vi "Layer Parameters Write Low Level.vi"(8 "Error In":errorcluster, 10 "Layer Information Cluster":T2 {"Deposition Method" items=["Front Electrode", "Electron Transport Layer", "Active Layer", "Hole Transport Layer", "Back Electrode", "Custom Layer"]; "Layer Type" items=["Front Electrode", "Electron Transport Layer", "Active Layer", "Hole Transport Layer", "Back Electrode", "Custom Layer"]}, 11 "Database Full Information In":T1 {"Database Write Information"."Layer Information Array"."Deposition Method" items=["Blade Coating", "Spin Coating", "Thermal Evaporation", "E-Beam Evaporation", "Sputtering", "Drop Casting", "Dip Coating", "Pulsed Laser Deposition", "Chemival Vapour Deposition", "Atomic Layer Deposition", "Spray Coating", "Screen Printing", "Electroplating", "Molecular Beam Epitaxy", "Custom Deposition"]; "Database Write Information"."Layer Information Array"."Layer Type" items=["Front Electrode", "Electron Transport Layer", "Active Layer", "Hole Transport Layer", "Back Electrode", "Custom Layer"]}) -> (0 "Error Out":errorcluster)   [LabVIEW 2020]
uses:
  Data Clusters/Layer Information Cluster.ctl
  Data Clusters/Database Information.ctl
  <vilib>/addons/database/Connection.llb/Conn ObjectReference.ctl
  <vilib>/addons/database/NI_Database_API.lvlib
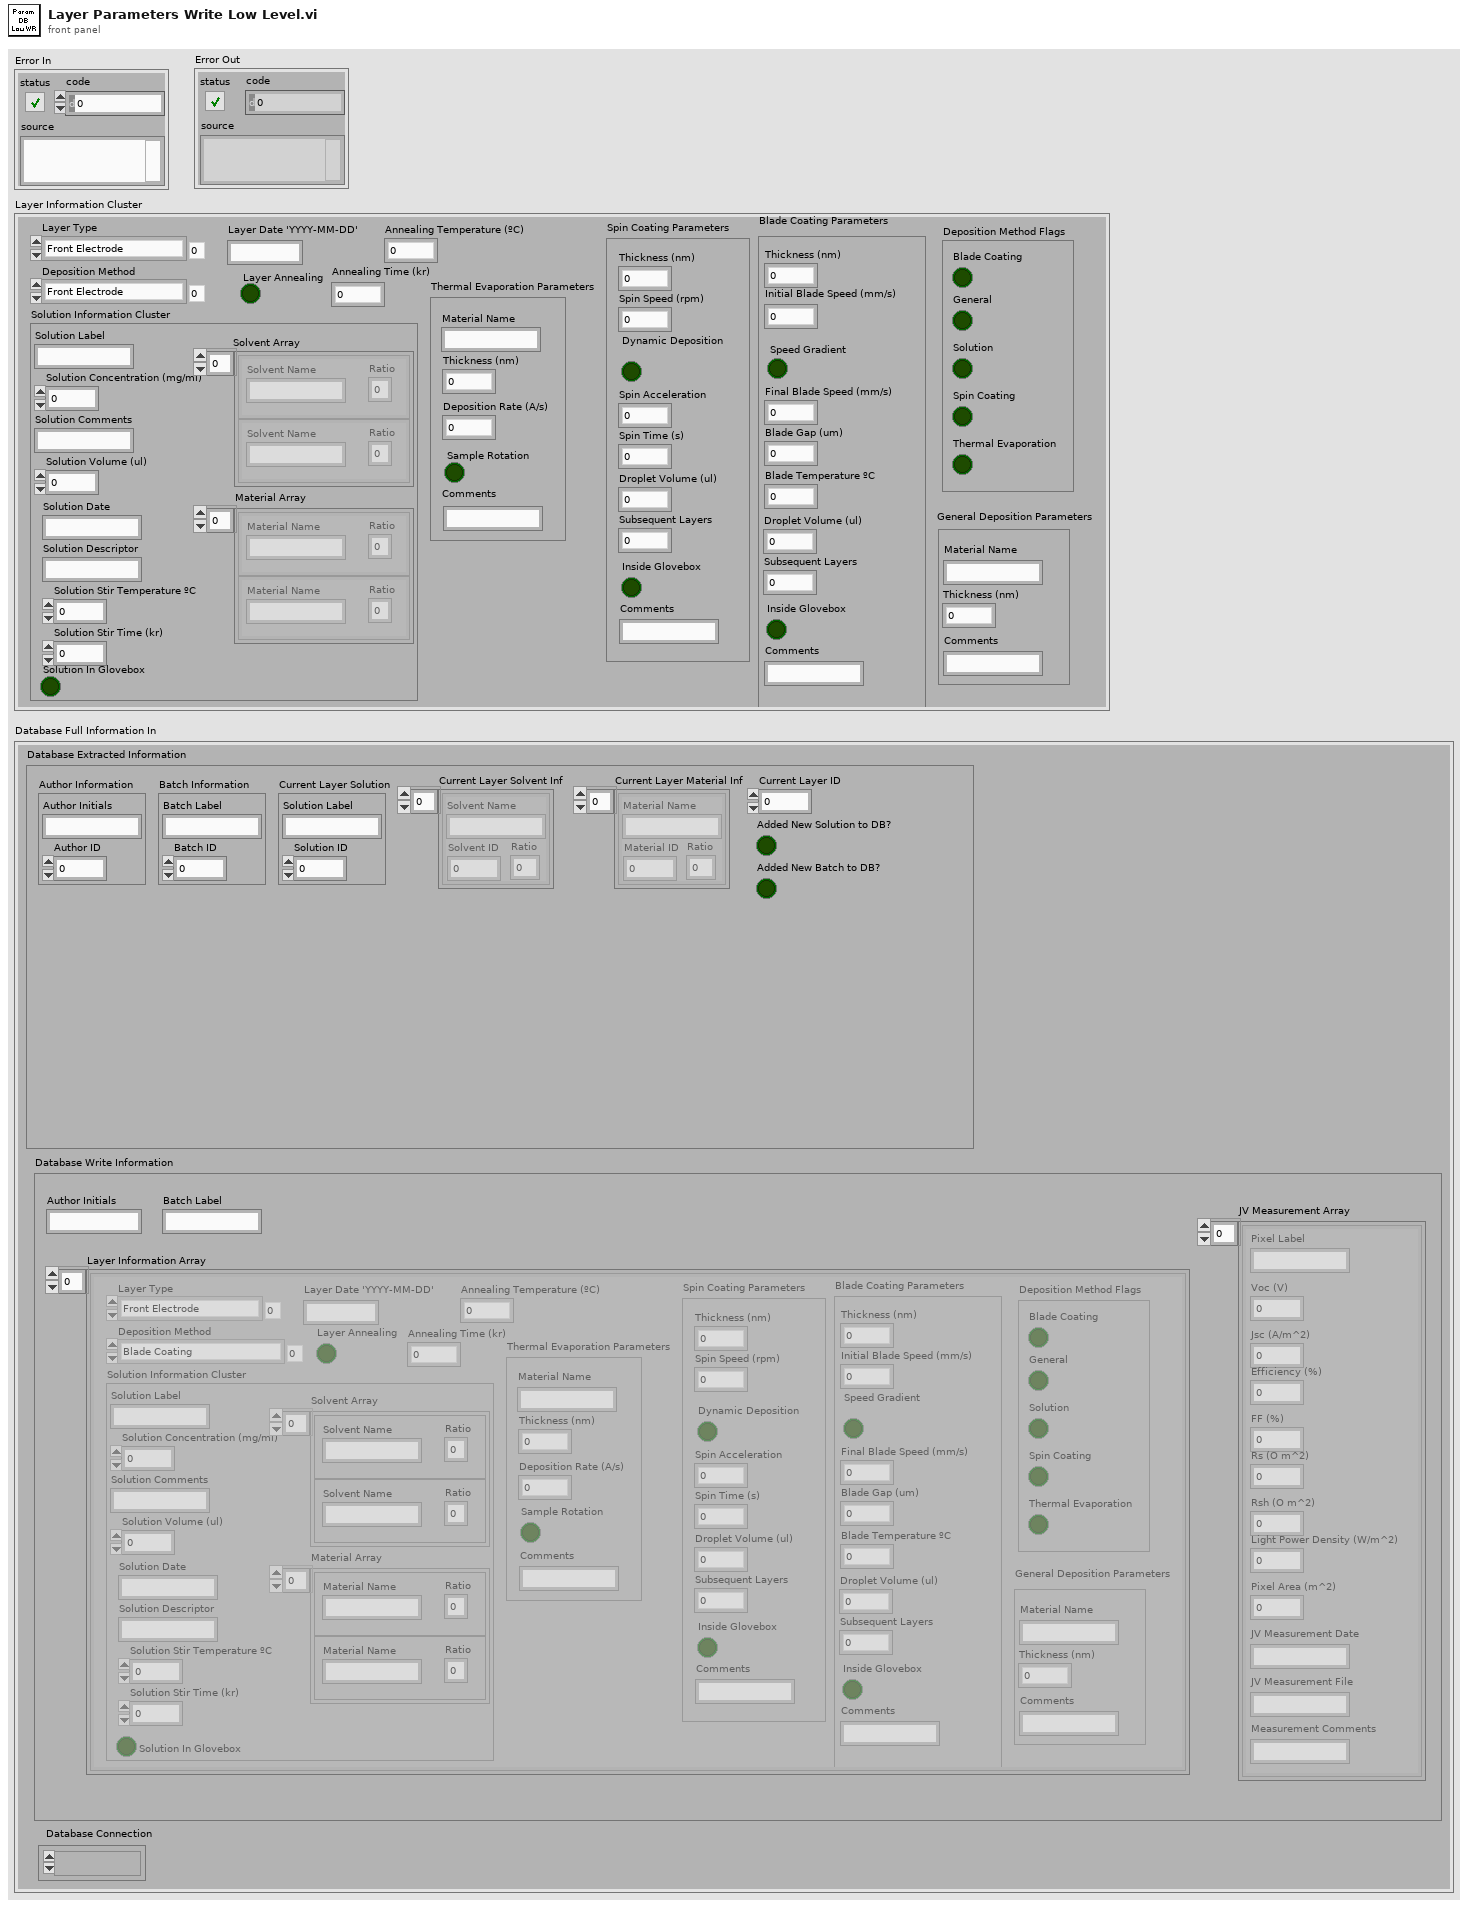
[diagram p1: front panel]
types:
  T1 = typedef "Database Information.ctl" = cluster{"Database Extracted Information":cluster{"Author Information":cluster{"Author Initials":string, "Author ID":i32}, "Batch Information":cluster{"Batch Label":string, "Batch ID":i32}, "Current Layer Solution":cluster{"Solution Label":string, "Solution ID":i32}, "Current Layer ID":i32, "Current Layer Solvent Inf":cluster{"Solvent Name":string, "Solvent ID":i32, "Ratio":dbl}[], "Current Layer Material Inf":cluster{"Material Name":string, "Material ID":i32, "Ratio":dbl}[], "Added New Solution to DB?":bool, "Added New Batch to DB?":bool}, "Database Write Information":cluster{"Author Initials":string, "Batch Label":string, "Layer Information Array":T2[], "JV Measurement Array":cluster{"Pixel Label":string, "Voc (V) ":dbl, "Jsc (A/m^2) ":dbl, "Efficiency (%)":dbl, "FF (%)":dbl, "Rs (O m^2)":dbl, "Rsh (O m^2)":dbl, "Light Power Density (W/m^2)":dbl, "Pixel Area (m^2)":dbl, "JV Measurement Date":string, "JV Measurement File":string, "Measurement Comments":string}[]}, "Database Connection":T3}
  T2 = typedef "Layer Information Cluster.ctl" = cluster{"Solution Information Cluster":cluster{"Solution Label":string, "Solution Concentration (mg/ml)":dbl, "Solution Comments ":string, "Solution Volume (ul) ":dbl, "Solution Date ":string, "Solution Descriptor ":string, "Solution Stir Temperature ºC ":dbl, "Solution Stir Time (kr) ":dbl, "Solution In Glovebox":bool, "Solvent Array":cluster{"Solvent Name":string, "Ratio":dbl}[], "Material Array":cluster{"Material Name":string, "Ratio":dbl}[]}, "Layer Type":u16, "Deposition Method":u16, "Layer Annealing":bool, "General Deposition Parameters":cluster{"Thickness (nm)":dbl, "Comments":string, "Material Name":string}, "Blade Coating Parameters":cluster{"Thickness (nm)":dbl, "Initial Blade Speed (mm/s)":dbl, "Speed Gradient":bool, "Final Blade Speed (mm/s)":dbl, "Blade Gap (um)":dbl, "Droplet Volume (ul)":dbl, "Subsequent Layers":dbl, "Inside Glovebox":bool, "Comments":string, "Blade Temperature ºC":dbl}, "Spin Coating Parameters":cluster{"Thickness (nm)":dbl, "Spin Speed (rpm)":dbl, "Dynamic Deposition":bool, "Spin Acceleration":dbl, "Spin Time (s)":dbl, "Droplet Volume (ul)":dbl, "Subsequent Layers":dbl, "Inside Glovebox":bool, "Comments":string}, "Thermal Evaporation Parameters":cluster{"Deposition Rate (A/s)":dbl, "Thickness (nm)":dbl, "Comments":string, "Material Name":string, "Sample Rotation":bool}, "Layer Date 'YYYY-MM-DD'":string, "Annealing Time (kr)":dbl, "Annealing Temperature (ºC)":dbl, "Deposition Method Flags":cluster{"Blade Coating":bool, "General ":bool, "Solution":bool, "Spin Coating":bool, "Thermal Evaporation":bool}}
  T3 = typedef "NI_Database_API.lvlib/Conn ObjectReference.ctl" = refnum<k1>
  T4 = enum16{"General Parameters", "Spin Coating", "Blade Coating", "Thermal Evaporation"}
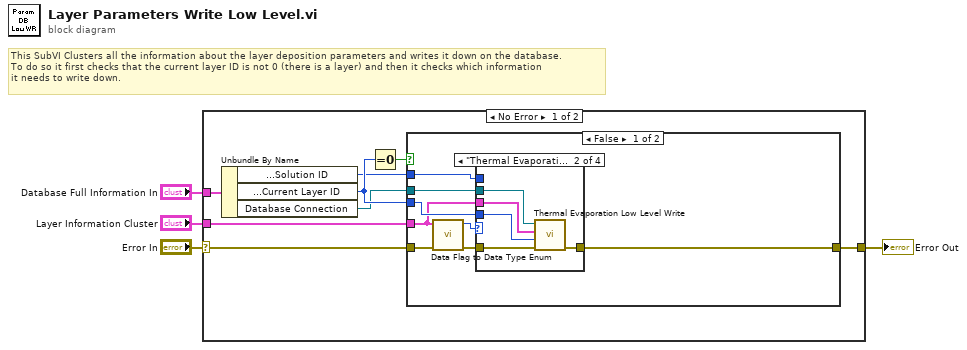
[diagram p0: block diagram]
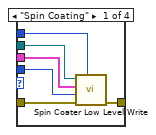
[diagram p2: hidden frame]
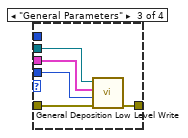
[diagram p3: hidden frame]
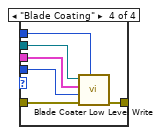
[diagram p4: hidden frame]
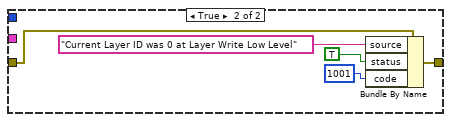
[diagram p5: hidden frame]
diagram:
  # "This SubVI Clusters all the information about the layer deposition parameters and writes it down on the database.\nTo do so it first checks that the current layer ID is not 0 (there is a layer) and then it checks which information \nit needs to write down."
  n1 = case shown="No Error" "Error In" {
    selector: "Error In" -> [w11 w48]
    tunnel: [w12 w48] -> w4
    tunnel: "Layer Information Cluster" -> [w10 _]
    tunnel: "Database Full Information In" -> [w8 _]
    frame No Error {
      n2 = Unbundle By Name(w8) -> ("Database Extracted Information.Current Layer Solution.Solution ID"=w6:i32, "Database Extracted Information.Current Layer ID"=w7:i32, "Database Connection"=w5:T3)
      n3 = Equal To 0?(x=w7) -> (x = 0?=w9:bool)
      n4 = case shown="False" w9 {
        tunnel: [w20 w45] -> w12
        tunnel: w5 -> [w19 _]
        tunnel: w11 -> [w16 w47]
        tunnel: w10 -> [w14 _]
        tunnel: w7 -> [w18 _]
        tunnel: w6 -> [w17 _]
        frame False {
          n5 = call "Data Flag to Data Type Enum.vi"("Error In"=w16, "Layer Information Cluster"=w14) -> ("Error Out"=w15:errorcluster, "Data Type"=w13:T4)  [unwired: 8 in]
          n6 = case shown="\"Thermal Evaporation\"" w13 {
            tunnel: [w26 w31 w36 w42] -> w20
            tunnel: w19 -> [w25 w30 w35 w41]
            tunnel: w15 -> [w24 w29 w34 w40]
            tunnel: w18 -> [w23 w28 w33 w39]
            tunnel: w14 -> [w22 w27 w32 w38]
            tunnel: w17 -> [w21 _ _ w37]
            frame "Spin Coating" {
              n7 = call "Spin Coater Low Level Write.vi"("Solution ID"=w21, "Error In"=w24, "Current Layer ID"=w23, "Layer Information Cluster"=w22, "Refnum in"=w25) -> ("Error Out"=w26:errorcluster)  [unwired: 5 in, 1 out]
            }
            frame "Thermal Evaporation" {
              n8 = call "Thermal Evaporation Low Level Write.vi"("Error In"=w29, "Current Layer ID"=w28, "Layer Information Cluster"=w27, "Refnum in"=w30) -> ("Error Out"=w31:errorcluster)  [unwired: 6 in, 1 out]
            }
            frame "General Parameters" {
              n9 = call "General Deposition Low Level Write.vi"("Error In"=w34, "Current Layer ID"=w33, "Layer Information Cluster"=w32, "Refnum in"=w35) -> ("Error Out"=w36:errorcluster)  [unwired: 6 in, 1 out]
            }
            frame "Blade Coating" {
              n10 = call "Blade Coater Low Level Write.vi"("Solution ID"=w37, "error in (no error)"=w40, "Current Layer ID"=w39, "Layer Information Cluster"=w38, "Refnum in"=w41) -> ("error out"=w42:errorcluster)  [unwired: 5 in, 1 out]
            }
          }
        }
        frame True {
          n11 = Bundle By Name(cluster=w47, "source"="Current Layer ID was 0 at Layer Write Low Level", "status"=TRUE, "code"=1001) -> (w45:errorcluster)
        }
      }
    }
    frame Error {
    }
  }
  "Error Out" <- w4
